vi "shippingWithout Color.vi"() -> ()   [LabVIEW 2012]
uses:
  <vilib>/Utility/NIReport.llb/NI_report.lvclass
  Global1.vi
  <vilib>/addons/database/Connection.llb/DB Tools Open Connec (Path).vi
  <vilib>/addons/_office/excel.llb/Excel Get Data (str).vi
  <vilib>/Utility/NIReport.llb/Excel/NI_Excel.lvclass
  <vilib>/addons/_office/NI_ReportGenerationToolkit.lvlib
  <vilib>/addons/database/NI_Database_API.lvlib
panel:
  out "String":string
  out "x+y":i32
  out "size(s)":i32
  out "error out":errorcluster
  out "error out 4":errorcluster
  out "String 3":string
  out "String 2":string
  in  "start (0, 0)":cluster{"start row":i32, "start column":i32}
  out "row":i32
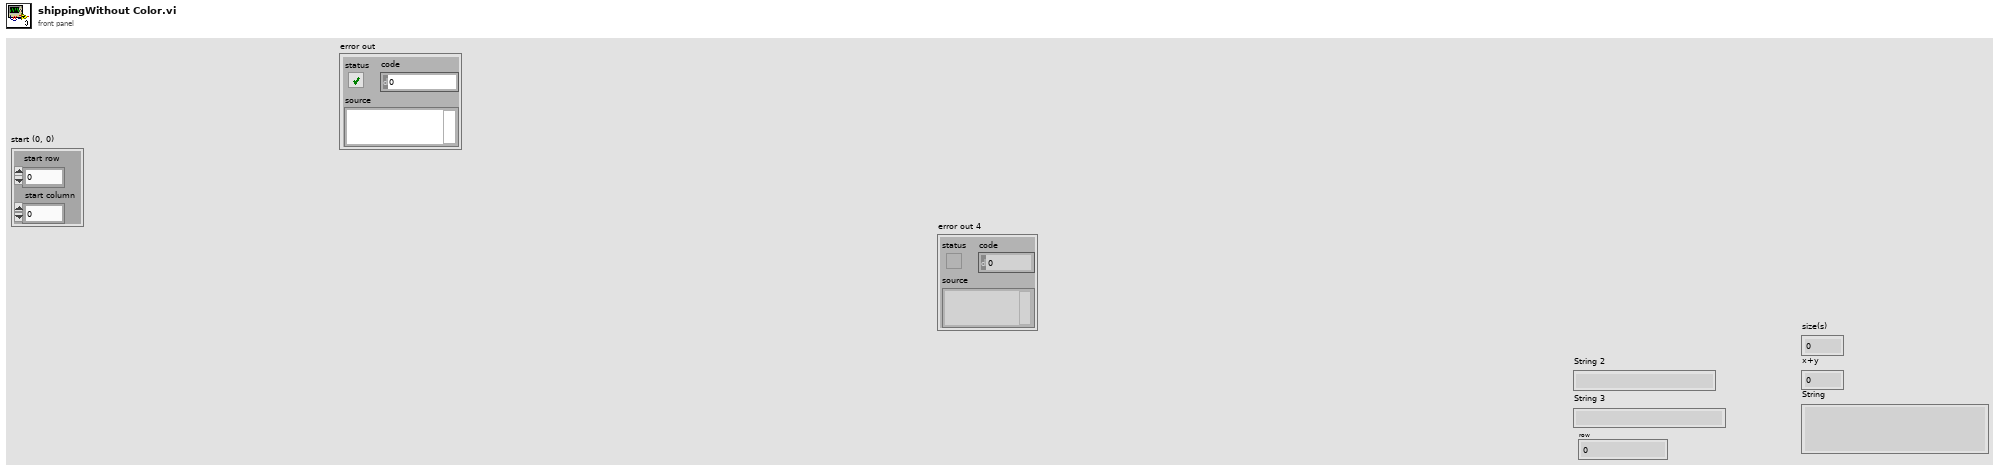
[diagram p1: front panel]
types:
  T1 = enum16{"Standard Report", "HTML", "Word", "Excel"}
  T2 = typedef "NI_Database_API.lvlib/Conn ObjectReference.ctl" = refnum<k1>
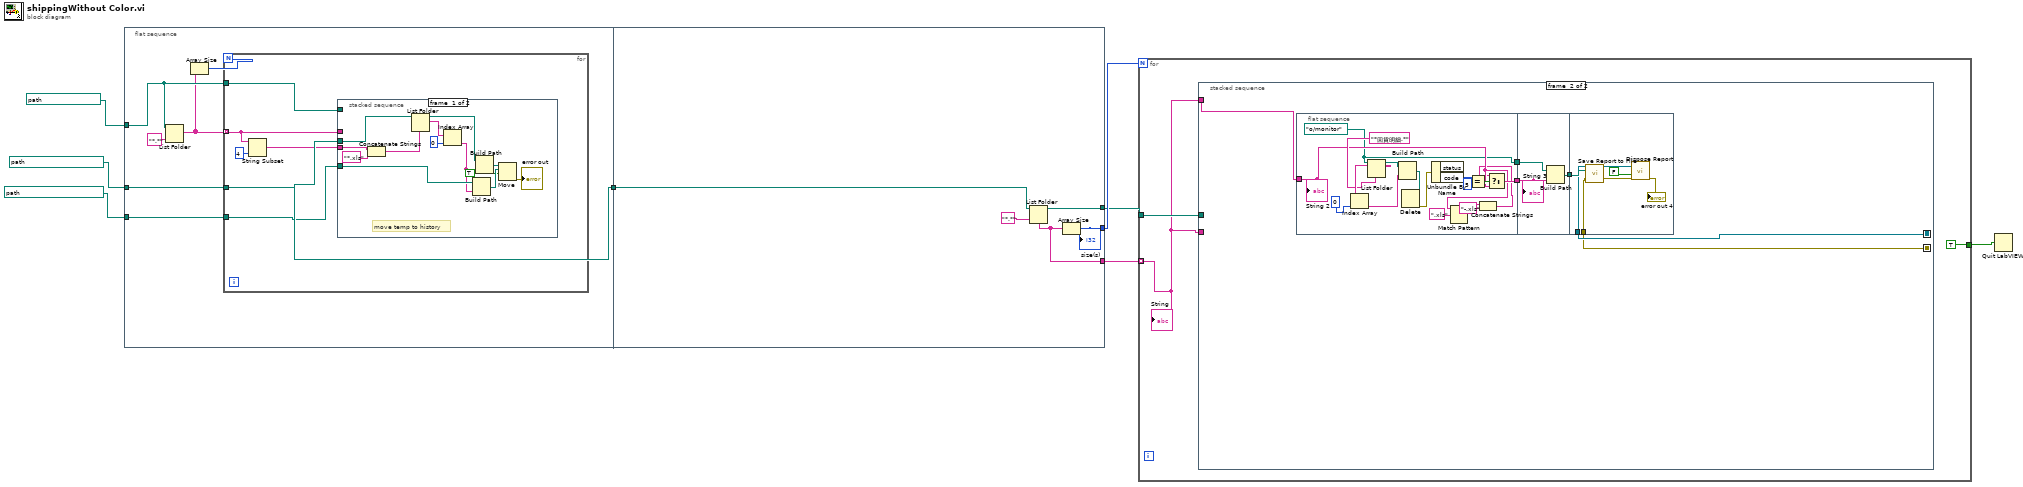
[diagram p0: block diagram]
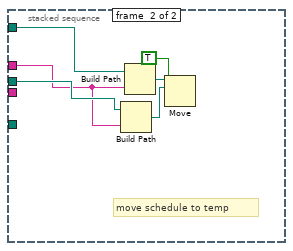
[diagram p2: hidden frame]
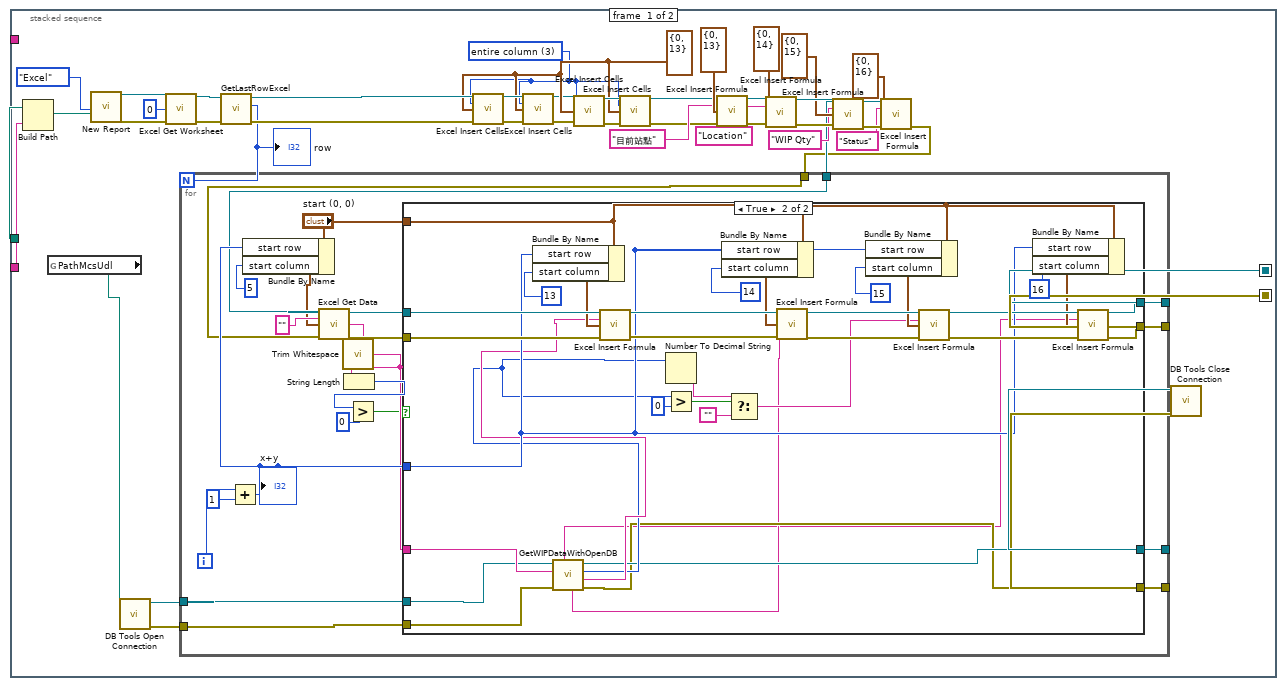
[diagram p3: hidden frame]
diagram:
  n1 = flat-sequence {
    tunnel: path "o:/monitor/回貨明細/temp" ("path") -> [w11]
    tunnel: [w11] -> w3
    tunnel: path "o:/monitor/回貨明細" ("path") -> [w13]
    tunnel: path "o:/monitor/回貨明細/history" ("path") -> [w12]
    tunnel: w3 -> [w43]
    tunnel: [w42] -> w5
    tunnel: [w41] -> w4
    tunnel: [w40] -> w2
    frame #0 {
      n2 = List Folder(path=w13, pattern="*.*") -> (filenames=w9:string[])  [unwired: 2 in, 3 out]
      n3 = Array Size(array=w9) -> (size(s)=w10:i32)
      n4 = for {
        N: w10 -> [_]
        tunnel: w13 -> [w20]
        tunnel: w12 -> [w19]
        tunnel: w11 -> [w18]
        tunnel: w9 -> [w15] mode=indexing
        n5 = String Subset(string=w15, length (rest)=4 ("length (rest)")) -> (substring=w16:string)  [unwired: 1 in]
        n6 = stacked-sequence {
          tunnel: w18 -> [w29 w36]
          tunnel: w19 -> [w32 _]
          tunnel: w20 -> [_ w37]
          tunnel: w16 -> [w24 _]
          tunnel: w15 -> [_ w34]
          frame #0 {
            # "move temp to history"
            n7 = Concatenate Strings(w24, "*.xls" ("pattern")) -> (w22:string)
            n8 = List Folder(path=w29, pattern=w22) -> (path out=w28:path, filenames=w27:string[])  [unwired: 2 in, 2 out]
            n9 = Index Array(array=w27, index=0) -> (element=w25:string)
            n10 = Build Path(base path=w32, name or relative path=w25) -> (appended path=w31:path)
            n11 = Build Path(base path=w28, name or relative path=w25) -> (appended path=w33:path)
            n12 = Move(source path=w33, 9:TRUE ("overwrite (F)"), 10:w31) -> (error out=→"error out":errorcluster)  [unwired: 2 in, 2 out]
          }
          frame #1 {
            # "move schedule to temp"
            n13 = Build Path(base path=w36, name or relative path=w34) -> (appended path=w38:path)
            n14 = Build Path(base path=w37, name or relative path=w34) -> (appended path=w39:path)
            n15 = Move(source path=w39, 9:TRUE ("overwrite (F)"), 10:w38) -> ()  [unwired: 2 in, 3 out]
          }
        }
      }
    }
    frame #1 {
      n16 = List Folder(path=w43, pattern="*.*") -> (path out=w41:path, filenames=w40:string[])  [unwired: 2 in, 2 out]
      n17 = Array Size(array=w40) -> (size(s)=w42:i32)
      "size(s)" <- w42
    }
  }
  n18 = for {
    N: w5 -> [_]
    tunnel: w4 -> [w47]
    tunnel: w2 -> [w46] mode=indexing
    tunnel: [TRUE] -> w1
    n19 = stacked-sequence {
      seq-local: [w69 _] -> [_ w153]
      seq-local: [w55 _] -> [_ w154]
      tunnel: w47 -> [w92 _]
      tunnel: w46 -> [w91 _]
      tunnel: w46 -> [_ w156]
      frame #0 {
        w62 = cluster{"row":i32, "column":i32} {"row"=0, "column"=13} ("start (0, 0)")
        w59 = u16 3 items=["shift cells right", "shift cells down", "entire row", "entire column"] ("mode (entire row)")
        n20 = Build Path(base path=w92, name or relative path=w91) -> (appended path=w90:path)
        n21 = global read "Global1.vi" "PathMcsUdl"() -> (w82:path)
        n22 = call <vilib>:"New Report.vi"("report type"=T1."Excel" ("Report Type"), "template (empty)"=w90) -> ("report out"=w88:refnum<class "NI_report.lvclass">, "error out"=w87:errorcluster)  [unwired: 12 in]
        n23 = call-poly <vilib>:"DB Tools Open Connection.vi"("connection information"=w82) -> ("error out"=w80:errorcluster, "connection reference"=w81:T2)  [unwired: 7 in]
        n24 = call <vilib>:"Excel Get Worksheet.vi"("report in"=w88, "worksheet index (0)"=0, "error in (no error)"=w87) -> ("report out"=w68:refnum<class "NI_report.lvclass">, "error out"=w67:errorcluster)  [unwired: 11 in]
        n25 = call "GetLastRowExcel.vi"("error in (no error)"=w67, "report in"=w68) -> ("error out"=w66:errorcluster, "row"=w50:i32, "report out"=w65:refnum<class "NI_report.lvclass">)  [unwired: 7 in]
        "row" <- w50
        n26 = call <vilib>:"Excel Insert Cells.vi"("report in"=w65, "mode (entire row)"=w59, "start (0, 0)"=w62, "error in (no error)"=w66) -> ("report out"=w64:refnum<class "NI_report.lvclass">, "error out"=w63:errorcluster)  [unwired: 10 in]
        n27 = call <vilib>:"Excel Insert Cells.vi"("report in"=w64, "mode (entire row)"=w59, "start (0, 0)"=w62, "error in (no error)"=w63) -> ("report out"=w61:refnum<class "NI_report.lvclass">, "error out"=w60:errorcluster)  [unwired: 10 in]
        n28 = call <vilib>:"Excel Insert Cells.vi"("report in"=w61, "mode (entire row)"=w59, "start (0, 0)"=w62, "error in (no error)"=w60) -> ("report out"=w86:refnum<class "NI_report.lvclass">, "error out"=w85:errorcluster)  [unwired: 10 in]
        n29 = call <vilib>:"Excel Insert Cells.vi"("report in"=w86, "mode (entire row)"=w59, "start (0, 0)"=w62, "error in (no error)"=w85) -> ("report out"=w52:refnum<class "NI_report.lvclass">, "error out"=w51:errorcluster)  [unwired: 10 in]
        n30 = call <vilib>:"Excel Insert Formula.vi"("report in"=w52, "formula"="目前站點", "start (0, 0)"=cluster{"row":i32, "column":i32} {"row"=0, "column"=13}, "error in (no error)"=w51) -> ("report out"=w79:refnum<class "NI_report.lvclass">, "error out"=w77:errorcluster)  [unwired: 10 in]
        n31 = call <vilib>:"Excel Insert Formula.vi"("report in"=w79, "formula"="Location", "start (0, 0)"=cluster{"row":i32, "column":i32} {"row"=0, "column"=14}, "error in (no error)"=w77) -> ("report out"=w78:refnum<class "NI_report.lvclass">, "error out"=w76:errorcluster)  [unwired: 10 in]
        n32 = call <vilib>:"Excel Insert Formula.vi"("report in"=w78, "formula"="WIP Qty", "start (0, 0)"=cluster{"row":i32, "column":i32} {"row"=0, "column"=15}, "error in (no error)"=w76) -> ("report out"=w58:refnum<class "NI_report.lvclass">, "error out"=w57:errorcluster)  [unwired: 10 in]
        n33 = call <vilib>:"Excel Insert Formula.vi"("report in"=w58, "formula"="Status", "start (0, 0)"=cluster{"row":i32, "column":i32} {"row"=0, "column"=16}, "error in (no error)"=w57) -> ("report out"=w49:refnum<class "NI_report.lvclass">, "error out"=w48:errorcluster)  [unwired: 10 in]
        n34 = for {
          N: w50 -> [_]
          tunnel: [w104] -> w69
          tunnel: [w97] -> w84
          tunnel: [w96] -> w83
          tunnel: w81 -> [w95]
          tunnel: w80 -> [w94]
          tunnel: [w105] -> w55
          tunnel: w49 -> [w102]
          tunnel: w48 -> [w103]
          i -> [w109]
          n35 = Add(x=w109, y=1) -> (x+y=w107:i32)
          "x+y" <- w107
          n36 = Bundle By Name(cluster="start (0, 0)", "start row"=w107, "start column"=5) -> (w110:cluster{"start row":i32, "start column":i32})
          n37 = call-poly <vilib>:"Excel Get Data.vi"("report in"=w102, "data type"="", "start (0, 0)"=w110, "error in (no error)"=w103) -> ("report out"=w113:refnum<class "NI_report.lvclass">, "data"=w99:string, "error out"=w112:errorcluster)  [unwired: 9 in]
          n38 = call <vilib>:"Trim Whitespace.vi"("string"=w99) -> ("trimmed string"=w98:string)  [unwired: 1 in]
          n39 = String Length(string=w98) -> (length=w101:i32)
          n40 = Greater?(x=w101, y=0) -> (0:w93:bool)
          n41 = case shown="True" w93 {
            tunnel: w113 -> [w118 w152]
            tunnel: w112 -> [w117 w151]
            tunnel: w107 -> [_ w133]
            tunnel: "start (0, 0)" -> [_ w132]
            tunnel: [w118 w131] -> w105
            tunnel: [w117 w130] -> w104
            tunnel: w98 -> [_ w127]
            tunnel: [w116 w124] -> w97
            tunnel: [w115 w123] -> w96
            tunnel: w95 -> [w116 w120]
            tunnel: w94 -> [w115 w119]
            frame False {
            }
            frame True {
              n42 = Bundle By Name(cluster=w132, "start row"=w133, "start column"=13) -> (w129:cluster{"start row":i32, "start column":i32})
              n43 = call "GetWIPDataWithOpenDB.vi"("error in (no error)"=w119, "Lotno"=w127, "connection reference"=w120) -> ("error out"=w123:errorcluster, "step"=w126:string, "data"=w125:i32, "connection reference 2"=w124:T2, "location"=w122:string, "status"=w121:string)  [unwired: 3 in]
              n44 = call <vilib>:"Excel Insert Formula.vi"("report in"=w152, "formula"=w126, "start (0, 0)"=w129, "error in (no error)"=w151) -> ("report out"=w147:refnum<class "NI_report.lvclass">, "error out"=w144:errorcluster)  [unwired: 10 in]
              n45 = Number To Decimal String(number=w125) -> (decimal integer string=w140:string)  [unwired: 1 in]
              n46 = Greater?(x=w125, y=0) -> (0:w139:bool)
              n47 = Bundle By Name(cluster=w132, "start row"=w133, "start column"=14) -> (w142:cluster{"start row":i32, "start column":i32})
              n48 = Select(t=w140, s=w139, f="") -> (s? t:f=w137:string)
              n49 = call <vilib>:"Excel Insert Formula.vi"("report in"=w147, "formula"=w122, "start (0, 0)"=w142, "error in (no error)"=w144) -> ("report out"=w146:refnum<class "NI_report.lvclass">, "error out"=w145:errorcluster)  [unwired: 10 in]
              n50 = Bundle By Name(cluster=w132, "start row"=w133, "start column"=15) -> (w143:cluster{"start row":i32, "start column":i32})
              n51 = call <vilib>:"Excel Insert Formula.vi"("report in"=w146, "formula"=w137, "start (0, 0)"=w143, "error in (no error)"=w145) -> ("report out"=w135:refnum<class "NI_report.lvclass">, "error out"=w134:errorcluster)  [unwired: 10 in]
              n52 = Bundle By Name(cluster=w132, "start row"=w133, "start column"=16) -> (w128:cluster{"start row":i32, "start column":i32})
              n53 = call <vilib>:"Excel Insert Formula.vi"("report in"=w135, "formula"=w121, "start (0, 0)"=w128, "error in (no error)"=w134) -> ("report out"=w131:refnum<class "NI_report.lvclass">, "error out"=w130:errorcluster)  [unwired: 10 in]
            }
          }
        }
        n54 = call <vilib>:"DB Tools Close Connection.vi"("error in (no error)"=w83, "connection reference"=w84) -> ()  [unwired: 5 in, 1 out]
      }
      frame #1 {
        n55 = flat-sequence {
          tunnel: [w159] -> w158
          tunnel: w156 -> [w161]
          tunnel: [w162] -> w157
          tunnel: w158 -> [w178]
          tunnel: w157 -> [w177]
          tunnel: [w176] -> w155
          tunnel: w155 -> [w181]
          tunnel: w154 -> [w180]
          tunnel: w153 -> [w179]
          frame #0 {
            w159 = path "o:/monitor" ("base path")
            n56 = List Folder(path=w159, pattern="*回貨明細.*") -> (path out=w173:path, filenames=w175:string[])  [unwired: 2 in, 2 out]
            n57 = Index Array(array=w175, index=0) -> (element=w172:string)
            n58 = Build Path(base path=w173, name or relative path=w172) -> (appended path=w170:path)
            n59 = Delete(path (use dialog)=w170) -> (error out=w169:errorcluster)  [unwired: 4 in, 2 out]
            n60 = Unbundle By Name(w169) -> ("code"=w168:i32)  [unwired: 1 out]
            n61 = Match Pattern(string=w161, regular expression=".xls") -> (match substring=w164:string)  [unwired: 1 in, 3 out]
            n62 = Equal?(x=w168, y=5) -> (x = y?=w166:bool)
            n63 = Concatenate Strings(w164, "-.xls" ("string")) -> (w160:string)
            n64 = Select(t=w160, s=w166, f=w161) -> (s? t:f=w162:string)
            "String 2" <- w161
          }
          frame #1 {
            n65 = Build Path(base path=w178, name or relative path=w177) -> (appended path=w176:path)
            "String 3" <- w177
          }
          frame #2 {
            n66 = call-dynamic "Save Report to File.vi"("report in"=w180, "report file path"=w181, "error in (no error)"=w179) -> ("report out"=w182:refnum<class "NI_report.lvclass">, "error out"=w183:errorcluster)  [unwired: 11 in]
            n67 = call-dynamic "Dispose Report.vi"("report in"=w182, "save changes? (F)"=FALSE, "error in (no error)"=w183) -> ("error out"=→"error out 4":errorcluster)  [unwired: 12 in]
          }
        }
      }
    }
    "String" <- w46
  }
  n68 = Quit LabVIEW(quit? (T)=w1) -> ()
